vi "DOConfigureClock_Speziale.vi"(0 "object in":refnum<class "AD2_DO_SDK.lvclass">, 1 "DO Trigger":T2, 2 "ClockSettings":T1(array[cluster]), 5 "error in (no error)":errorcluster) -> (14 "object out":refnum<class "AD2_DO_SDK.lvclass">, 19 "error out":errorcluster)   [LabVIEW 2024, in "AD2_DO_SDK.lvclass"]
uses:
  AD2_DO_SDK.lvclass
  DOTrigger.ctl
  AD2_WFG_SDK_class/AD2TriggerSources.ctl
  AD2_DO_SDK.lvclass/AD2_DO_SDK.ctl
  AD2_SDK_class/AD2_SDK.lvclass
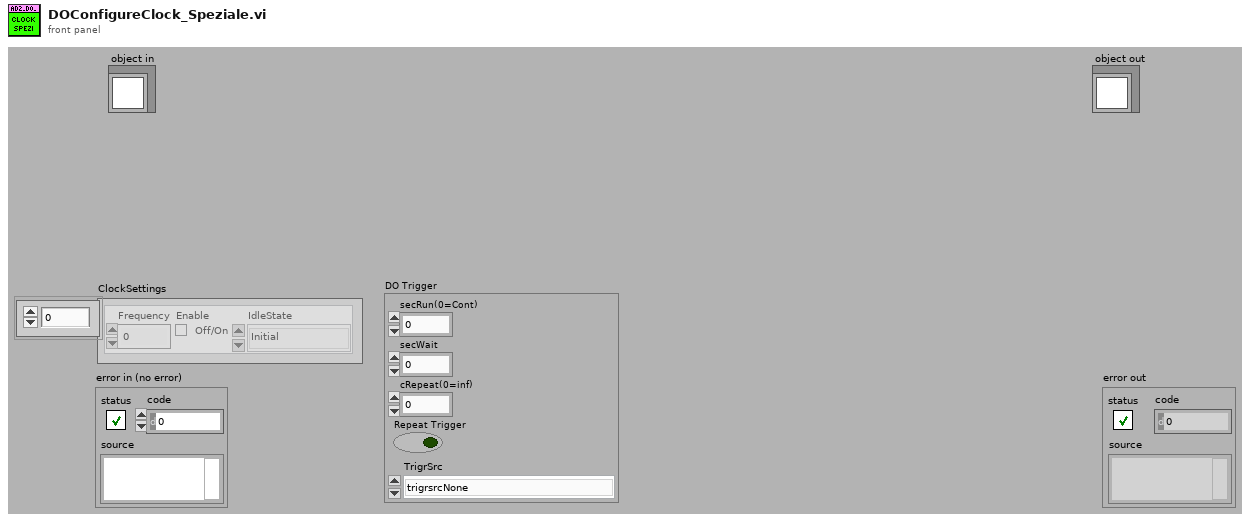
[diagram p1: front panel]
types:
  T1 = cluster{"Frequency":dbl, "Enable":bool, "IdleState":enum16{"Initial", "Low", "High", "Z"}}[]
  T2 = typedef "AD2_DO_SDK.lvclass/DOTrigger.ctl" = cluster{"secRun(0=Cont)":dbl, "secWait":dbl, "cRepeat(0=inf)":i32, "Repeat Trigger":bool, "TrigrSrc":T3}
  T3 = typedef "AD2_SDK.lvclass/AD2TriggerSources.ctl" = enum8{"trigrsrcNone", "trigsrcPC", "trigsrcDetectorAnalogIn", "trigsrcDetectorDigitalIn", "trigsrcAnalogIn", "trigsrcDigitalIn", "trigsrcDigitalOut", "trigsrcAnalogOut1", "trigsrcAnalogOut2", "trigsrcAnalogOut3", "trigsrcAnalogOut4", "trigsrcExternal1", "trigsrcExternal2", "trigsrcExternal3", "trigsrcExternal4", ""}
  T4 = cluster{"NoHighBits":u32, "NoLowBits":u32, "NoInitialBits":u32, "Start High":bool}
  T5 = typedef "AD2_DO_SDK.lvclass/DOSingleCh.ctl" = cluster{"Ch Index":i32, "Enable":bool, "Clock DIvider":u32, "Type":i32, "DigitalOutOutput":u16, "IdleState":u16, "CounterData":cluster{"NoHighBits":u32, "NoLowBits":u32, "NoInitialBits":u32, "Start High":bool}, "Custom Data":cluster{"countOfBits":u32, "rgBits":u8[]}}
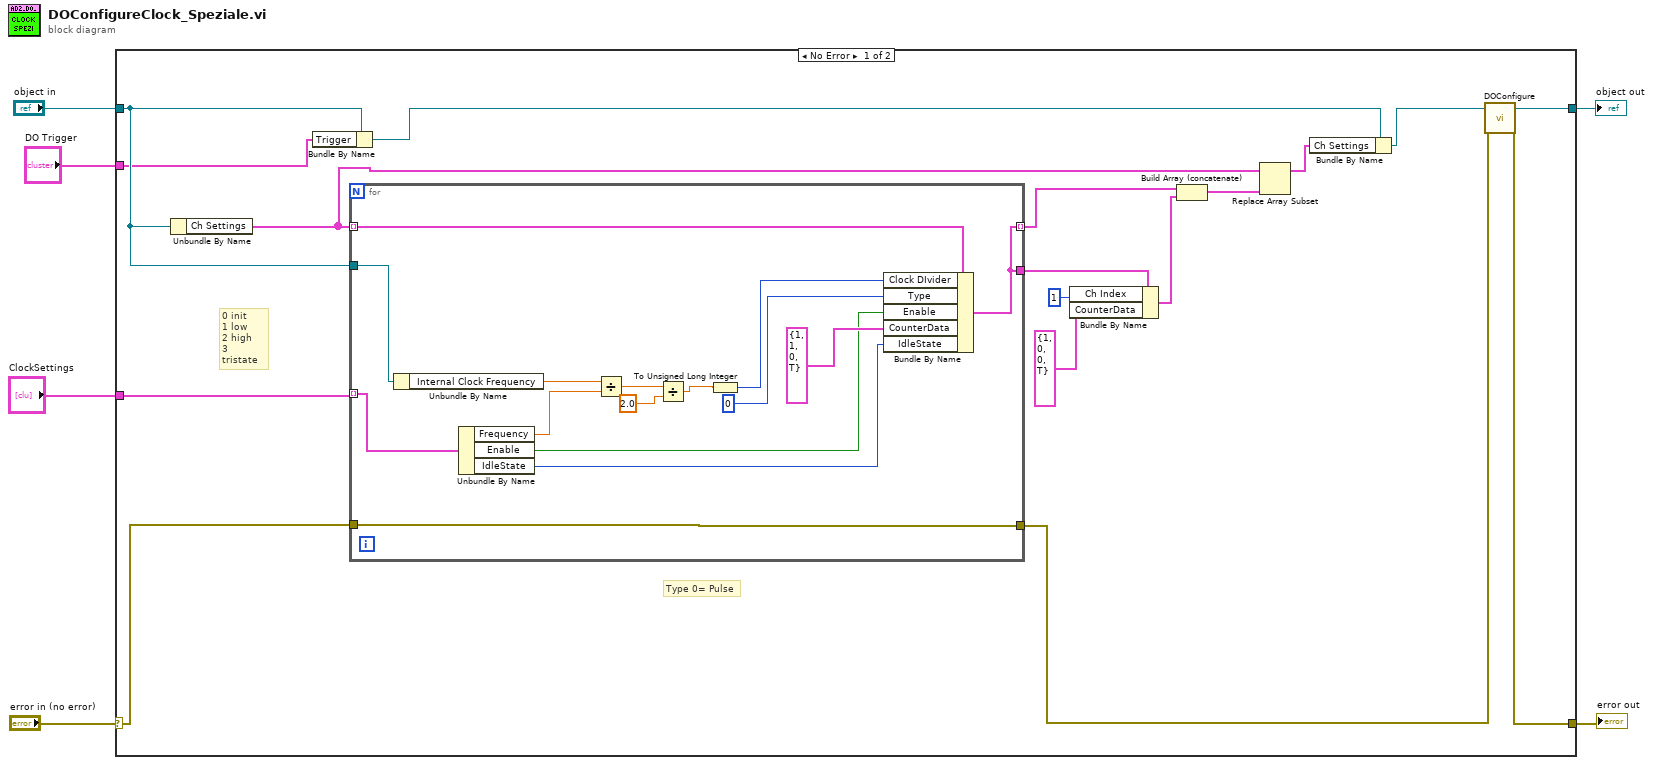
[diagram p0: block diagram]
diagram:
  n1 = case shown="No Error" "error in (no error)" {
    selector: "error in (no error)" -> [w19 w40]
    tunnel: [w23 w40] -> w5
    tunnel: [w22 w39] -> w3
    tunnel: "object in" -> [w17 w39]
    tunnel: "DO Trigger" -> [w16 _]
    tunnel: "ClockSettings" -> [w15 _]
    frame No Error {
      # "0 init\n1 low\n2 high\n3 tristate"
      # "Type 0= Pulse"
      n2 = Unbundle By Name(w17) -> ("Ch Settings"=w14:T5[])
      n3 = Bundle By Name(cluster=w17, "Trigger"=w16) -> (w18:refnum<class "AD2_DO_SDK.lvclass">)
      n4 = for {
        tunnel: w14 -> [w33] mode=indexing
        tunnel: [w24] -> w13 mode=indexing
        tunnel: w19 -> [w29]
        tunnel: [w29] -> w20
        tunnel: w17 -> [w38]
        tunnel: w15 -> [w28] mode=indexing
        tunnel: [w24] -> w11
        n5 = Unbundle By Name(w38) -> ("Internal Clock Frequency"=w37:dbl)
        n6 = Unbundle By Name(w28) -> ("Frequency"=w27:dbl, "Enable"=w26:bool, "IdleState"=w25:enum16{"Initial", "Low", "High", "Z"})
        n7 = Divide(x=w37, y=w27) -> (x/y=w31:dbl)
        n8 = Divide(x=w31, y=2.0) -> (x/y=w30:dbl)
        n9 = To Unsigned Long Integer(number=w30) -> (unsigned 32bit integer=w36:u32)
        n10 = Bundle By Name(cluster=w33, "Clock DIvider"=w36, "Type"=0, "Enable"=w26, "CounterData"=T4 {"NoHighBits"=1, "NoLowBits"=1, "NoInitialBits"=0, "Start High"=TRUE}, "IdleState"=w25) -> (w24:T5)
      }
      n11 = Bundle By Name(cluster=w11, "Ch Index"=1, "CounterData"=T4 {"NoHighBits"=1, "NoLowBits"=0, "NoInitialBits"=0, "Start High"=TRUE}) -> (w7:T5)
      n12 = Build Array (concatenate)(w13, w7) -> (w8:T5[])
      n13 = Replace Array Subset(array=w14, new element=w8) -> (w12:T5[])  [unwired: 1 in]
      n14 = Bundle By Name(cluster=w18, "Ch Settings"=w12) -> (w21:refnum<class "AD2_DO_SDK.lvclass">)
      n15 = call-dynamic "DOConfigure.vi"("object in"=w21, "error in (no error)"=w20) -> ("object out"=w22:refnum<class "AD2_DO_SDK.lvclass">, "error out"=w23:errorcluster)  [unwired: 16 in]
    }
    frame Error {
    }
  }
  "error out" <- w5
  "object out" <- w3
